vi "Translate Aliased Endpoint.vi"(10 "Alias Mapping":T1, 11 "Endpoint in":string) -> (3 "Endpoint out":string)   [LabVIEW 2017, in "Routing and Faulting System Explorer.lvlib"]
uses:
  Routing and Faulting System Explorer.lvlib
  Shared/Alias Mapping.ctl
  Shared/Routing and Faulting Shared.lvlib
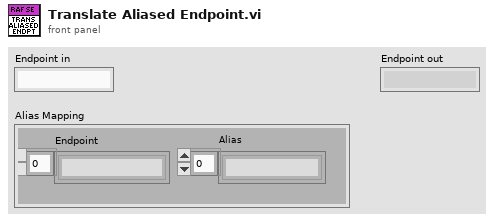
[diagram p1: front panel]
types:
  T1 = typedef "Routing and Faulting Shared.lvlib/Alias Mapping.ctl" = cluster{"Endpoint":string[], "Alias":string[]}
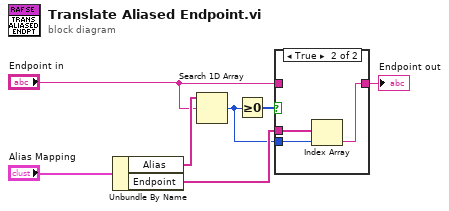
[diagram p0: block diagram]
diagram:
  n1 = Unbundle By Name("Alias Mapping") -> ("Alias"=w5:string[], "Endpoint"=w6:string[])
  n2 = Search 1D Array(1D array=w5, element="Endpoint in") -> (index of element=w2:i32)  [unwired: 1 in]
  n3 = Greater Or Equal To 0?(x=w2) -> (x >= 0?=w1:bool)
  n4 = case shown="True" w1 {
    tunnel: w6 -> [_ w11]
    tunnel: w2 -> [_ w10]
    tunnel: [w8 w9] -> w7
    tunnel: "Endpoint in" -> [w8 _]
    frame False {
    }
    frame True {
      n5 = Index Array(array=w11, index=w10) -> (element=w9:string)
    }
  }
  "Endpoint out" <- w7
